vi "Reset.vi"(8 "error in (no error)":errorcluster, 11 "VISA resource name":refnum<visa-resource-name>) -> (0 "error out":errorcluster, 3 "VISA resource name out":refnum<visa-resource-name>)   [LabVIEW 2021, in "Keithley 2200 Series.lvlib"]
doc: "Resets the instrument and then sends a set of default setup commands to the instrument.\n\nNote:\nRecommended waiting 4 seconds to run the next command."
uses:
  <instrlib>/Keithley 2200 Series/Keithley 2200 Series.lvlib
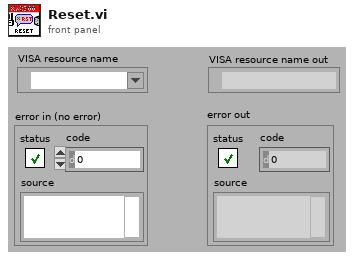
[diagram p1: front panel]
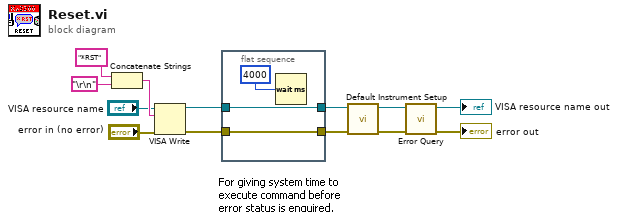
[diagram p0: block diagram]
diagram:
  n1 = Concatenate Strings("*RST" ("write buffer"), "\r\n" ("End of Line Constant")) -> (w6:string)
  n2 = VISA Write(VISA resource name="VISA resource name", write buffer=w6, error in (no error)="error in (no error)") -> (VISA resource name out=w13:refnum<visa-resource-name>, error out=w12:errorcluster)  [unwired: 1 out]
  n3 = flat-sequence {
    tunnel: w13 -> [w15]
    tunnel: w12 -> [w14]
    tunnel: [w15] -> w11
    tunnel: [w14] -> w8
    frame #0 {
      n4 = Wait (ms)(milliseconds to wait=u32 4000) -> ()  [unwired: 1 out]
    }
  }
  n5 = call <instrlib>:"Default Instrument Setup.vi"("error in (no error)"=w8, "VISA resource name"=w11) -> ("error out"=w7:errorcluster, "VISA resource name out"=w9:refnum<visa-resource-name>)  [unwired: 8 out]
  n6 = call <instrlib>:"Error Query.vi"("error in (no error)"=w7, "VISA resource name"=w9) -> ("error out"=→"error out":errorcluster, "VISA resource name out"=→"VISA resource name out":refnum<visa-resource-name>)  [unwired: 8 out]
